vi "Test 3.vi"(8 "error in (no error)":errorcluster, 11 "Test Case In":refnum<class "Tests.lvclass">) -> (0 "error out":errorcluster, 3 "Test Case Out":refnum<class "Tests.lvclass">)   [LabVIEW 2021, in "Tests.lvclass"]
uses:
  Tests.lvclass
  C:/Program Files (x86)/National Instruments/LabVIEW 2021/vi.lib/Astemes/LUnit/Test Case.lvclass
  <vilib>/Astemes/LUnit/Test Case.lvclass/Test Case.ctl
  4993e8ee-a06a-463a-9684-69129f64d5ce.vi
  <vilib>/Astemes/LUnit/Append Pass Result.vi
  <vilib>/Astemes/LUnit/Append Fail Result.vi
  <vilib>/Astemes/LUnit/Describe Comparison.vi
  <vilib>/Astemes/LUnit/Compare Variants.vi
  <vilib>/Astemes/LUnit/Variant to string.vi
  <vilib>/Utility/Data Type/Get Type Information.vi
  <vilib>/Utility/LVClass/Get LV Class Name.vi
  Tests.lvclass/Tests.ctl
  Proto/Maze.lvclass
  Beam/Beam.lvclass
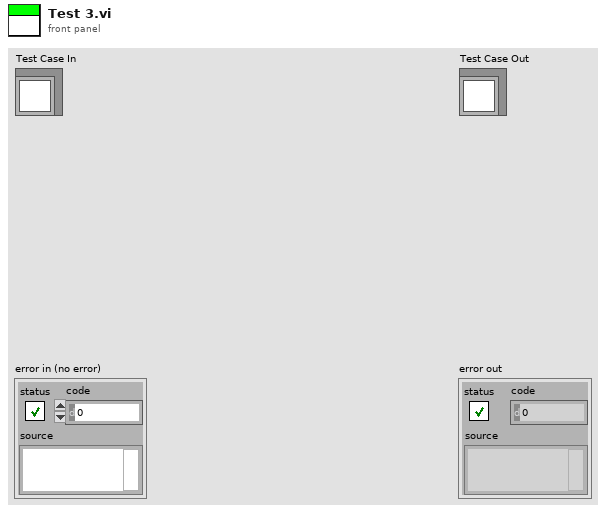
[diagram p1: front panel]
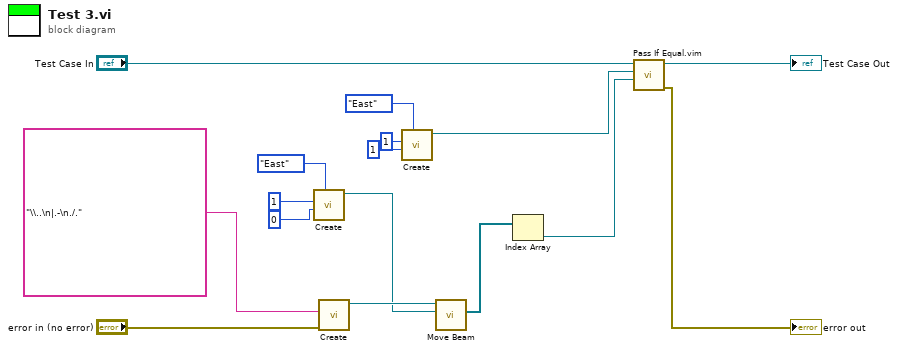
[diagram p0: block diagram]
diagram:
  n1 = call "Create.vi"("Direction"=enum16{"North", "East", "South", "West"}."East", "Col"=0, "Row"=1) -> ("Beam"=w8:refnum<class "Beam.lvclass">)  [unwired: 7 in, 1 out]
  n2 = call "Create.vi"("error in (no error)"="error in (no error)", "Input"="\\..\n|.-\n./.") -> ("Proto"=w12:refnum<class "Maze.lvclass">)  [unwired: 8 in, 1 out]
  n3 = call "Create.vi"("Direction"=enum16{"North", "East", "South", "West"}."East", "Col"=1, "Row"=1) -> ("Beam"=w2:refnum<class "Beam.lvclass">)  [unwired: 7 in, 1 out]
  n4 = call "Move Beam.vi"("Beam"=w8, "Maze In"=w12) -> ("Beams"=w5:refnum<class "Beam.lvclass">[])  [unwired: 8 in, 1 out]
  n5 = Index Array(array=w5) -> (element=w4:refnum<class "Beam.lvclass">)  [unwired: 1 in]
  n6 = call "Pass If Equal.vim"("Actual"=w4, "Expected"=w2, "LUnit Test Case In"="Test Case In") -> ("error out"=→"error out":errorcluster, "LUnit Test Case Out"=→"Test Case Out":refnum<class "Tests.lvclass">)  [unwired: 7 in]
